vi "Add Database RTM.vi"(8 "error in":errorcluster, 11 "Node Ptr":u64 format="%.0x") -> (0 "error out":errorcluster)   [LabVIEW 2020, in "Communication Bus Template System Explorer.lvlib"]
doc: "This VI runs when the Add Database run-time menu is chosen. It allows the user to choose a database file and rename the database if they want a name other than the file name."
uses:
  Communication Bus Template System Explorer.lvlib
  Types/Path Control.ctl
  Types/Browse Button.ctl
  Shared/Constants.vi
  <vilib>/NI VeriStand/Custom Device API/Set Item Property (Path).vi
  Shared/Communication Bus Template Shared.lvlib
  <vilib>/NI VeriStand/Custom Device Tools/Custom Device Utility Library/Custom Device Utility Library.lvlib
  <vilib>/NI VeriStand/Custom Device API/Custom Device API.lvlib
panel:
  in  "Path":T1
  in  "Database Name":string
  in  "Help":bool
  in  "Cancel":bool
  in  "OK":bool
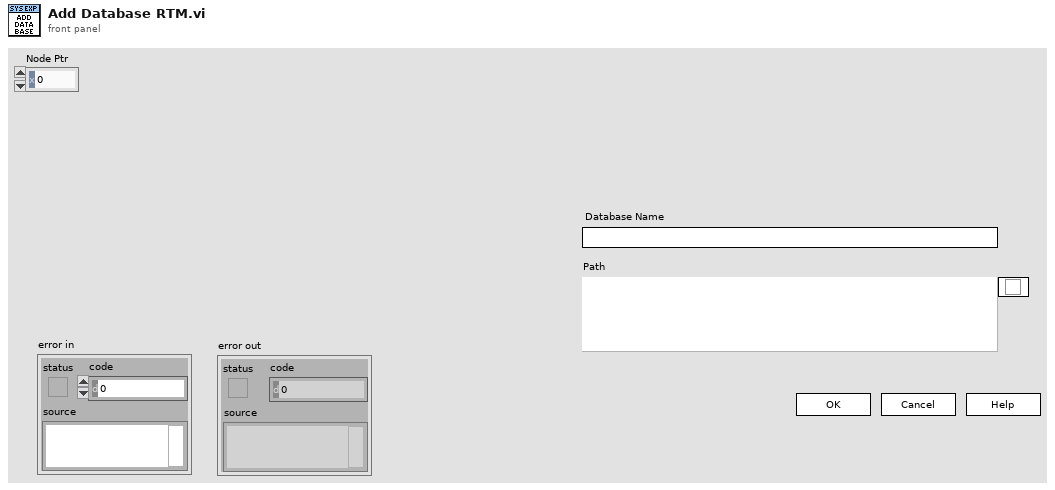
[diagram p1: front panel]
types:
  T1 = typedef "Communication Bus Template System Explorer.lvlib/Path Control.ctl" = cluster{"Path":path, "Browse":T2}
  T2 = typedef "Communication Bus Template System Explorer.lvlib/Browse Button.ctl" = bool
  T3 = cluster{"Database Name":string, "Database Path":path, "Node Ptr":u64}
  T4 = typedef "Custom Device API.lvlib/Custom Device Item Ref.ctl" = u64
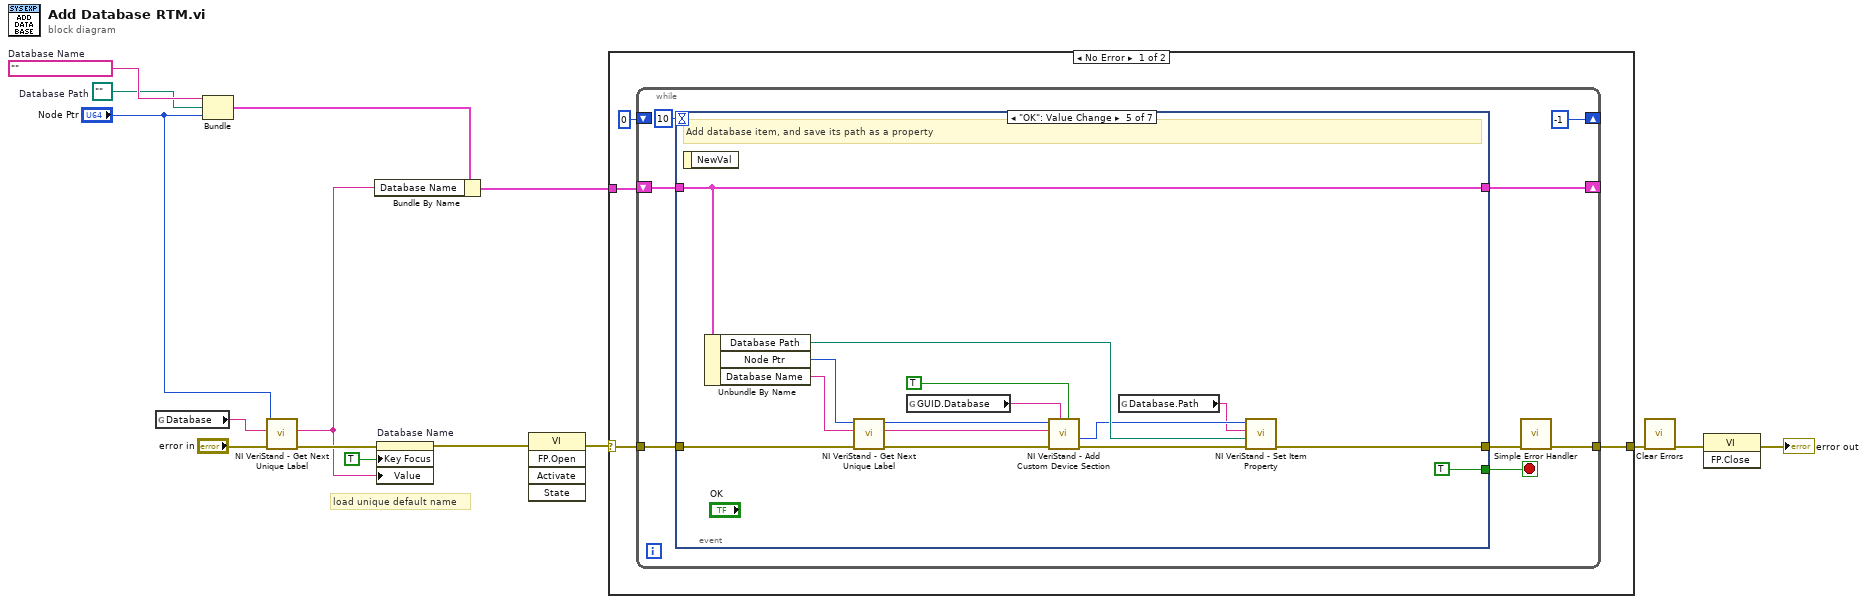
[diagram p0: block diagram]
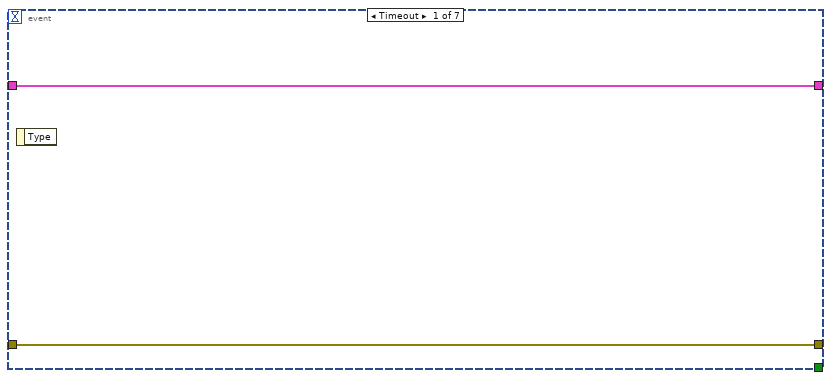
[diagram p2: hidden frame]
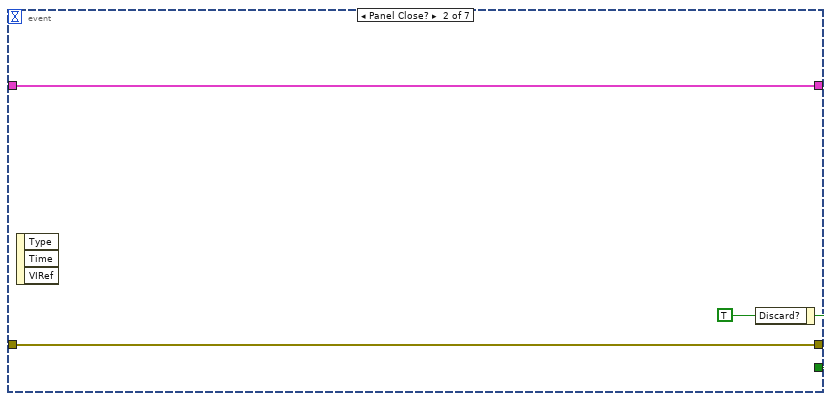
[diagram p3: hidden frame]
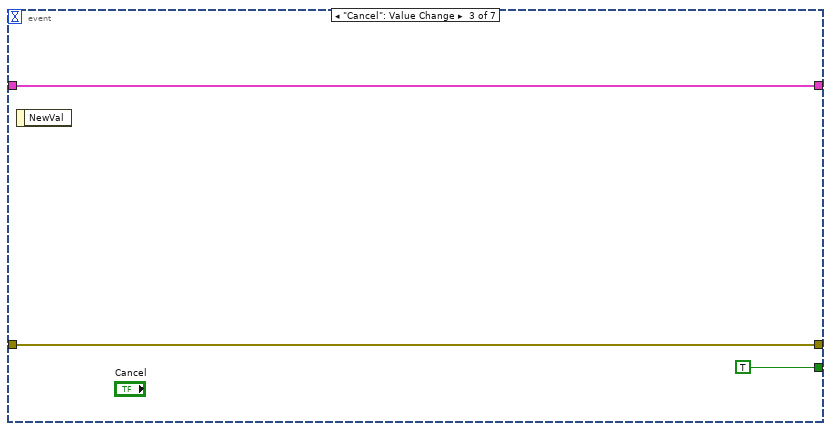
[diagram p4: hidden frame]
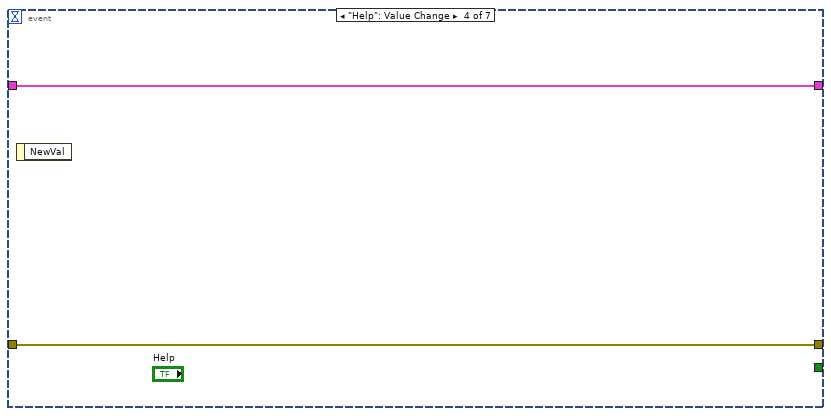
[diagram p5: hidden frame]
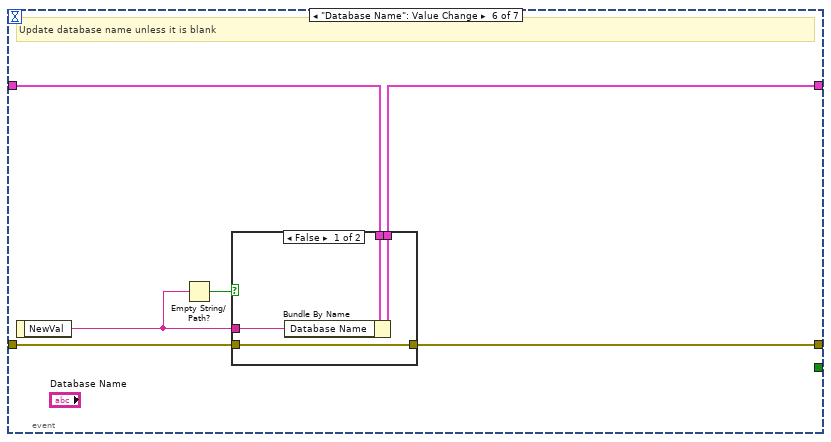
[diagram p6: hidden frame]
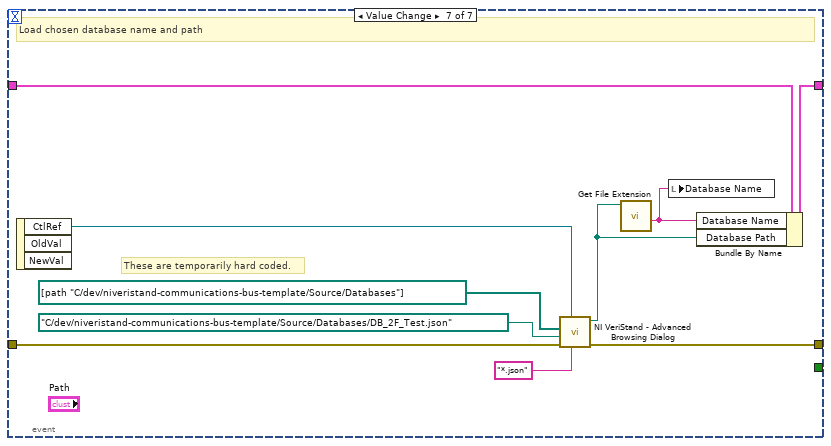
[diagram p8: hidden frame]
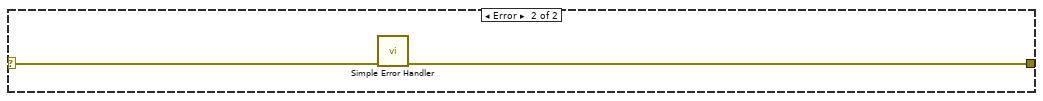
[diagram p9: hidden frame]
diagram:
  w1 = path ""  # Database Path
  w2 = ""  # Database Name
  # "load unique default name"
  n1 = global read "Constants.vi" "Database"() -> (w5:string)
  n2 = Bundle("Database Name"=w2, "Database Path"=w1, "Node Ptr"="Node Ptr") -> (w4:T3)  [unwired: 1 in]
  n3 = call <vilib>:"NI VeriStand - Get Next Unique Label.vi"("error in (no error)"="error in", "Label"=w5, "Parent Ref in"="Node Ptr") -> ("error out"=w7:errorcluster, "Label out"=w6:string)  [unwired: 5 in, 2 out]
  n4 = Bundle By Name(cluster=w4, "Database Name"=w6) -> (w13:T3)
  n5 = property on="Database Name" class="Str"(error in=w7, "Key Focus"=TRUE, "Value"=w6) -> (error out=w12:errorcluster)  [unwired: 1 in, 1 out]
  n6 = invoke class="VI" method="FP.Open"(error in=w12) -> (error out=w11:errorcluster)  [unwired: 4 in, 4 out]
  n7 = case shown="No Error" w11 {
    selector: w11 -> [w19 w76]
    tunnel: [w18 w75] -> w14
    tunnel: w13 -> [w16 _]
    frame No Error {
      n8 = while {
        tunnel: w19 -> [w27]
        tunnel: [w25] -> w18
        shift-right: [-1] -> _
        shift-left: 0 -> [_]
        shift-right: [w21] -> _
        shift-left: w16 -> [w22]
        stop <- w24 stop-if-true
        n9 = event shown="[4] \"OK\": Value Change" {
          selector: _ -> [_ _ _ _ _ _ _]
          dyn-events: _ -> [_ _ _ _ _ _ _]
          timeout: 10 -> [_ _ _ _ _ _ _]
          tunnel: [w29 w32 w34 w37 w39 w57 w69] -> w26
          tunnel: w27 -> [w29 w32 w34 w37 w48 w58 w73]
          tunnel: [_ w31 TRUE ("Discard?") _ TRUE ("Discard?") _ _] -> w24
          tunnel: w22 -> [w28 w30 w33 w36 w45 w54 w67]
          tunnel: [w28 w30 w33 w36 w45 w53 w68] -> w21
          event Timeout {
            n10 = event-data() -> ()  [unwired: 1 in, 1 out]
          }
          event Panel Close? {
            w31 = TRUE ("Discard?")
            n11 = event-data() -> ()  [unwired: 1 in, 3 out]
            n12 = event-data("Discard?"=w31) -> ()  [unwired: 1 in, 1 out]
          }
          event "Cancel": Value Change {
            n13 = event-data() -> ()  [unwired: 1 in, 1 out]
          }
          event "Help": Value Change {
            n14 = event-data() -> ()  [unwired: 1 in, 1 out]
          }
          event "OK": Value Change {
            # "Add database item, and save its path as a property"
            n15 = event-data() -> ()  [unwired: 1 in, 1 out]
            n16 = Unbundle By Name(w45) -> ("Database Path"=w41:path, "Node Ptr"=w44:u64, "Database Name"=w43:string)
            n17 = call <vilib>:"NI VeriStand - Get Next Unique Label.vi"("error in (no error)"=w48, "Label"=w43, "Parent Ref in"=w44) -> ("error out"=w49:errorcluster, "Label out"=w46:string, "Parent Ref dup"=w47:T4)  [unwired: 5 in, 1 out]
            n18 = global read "Constants.vi" "GUID.Database"() -> (w50:string)
            n19 = call <vilib>:"NI VeriStand - Add Custom Device Section.vi"("Highlight? (F)"=TRUE, "GUID (Default Section)"=w50, "error in (no error)"=w49, "Section Name"=w46, "Parent Ref in"=w47) -> ("error out"=w42:errorcluster, "Section Ptr"=w40:T4)  [unwired: 3 in, 2 out]
            n20 = global read "Constants.vi" "Database.Path"() -> (w38:string)
            n21 = call-poly <vilib>:"NI VeriStand - Set Item Property.vi"("error in (no error)"=w42, "Value"=w41, "Property Name"=w38, "Item Ref in"=w40) -> ("error out"=w39:errorcluster)  [unwired: 5 in, 2 out]
          }
          event "Database Name": Value Change {
            # "Update database name unless it is blank"
            n22 = event-data() -> ("NewVal"=w55:string)  [unwired: 1 in]
            n23 = Empty String/Path?(string/path=w55) -> (empty?=w56:bool)
            n24 = case shown="False" w56 {
              tunnel: w58 -> [w62 w64]
              tunnel: w55 -> [w60 _]
              tunnel: [w62 w64] -> w57
              tunnel: w54 -> [w61 w63]
              tunnel: [w59 w63] -> w53
              frame False {
                n25 = Bundle By Name(cluster=w61, "Database Name"=w60) -> (w59:T3)
              }
              frame True {
              }
            }
          }
          event Value Change {
            # "These are temporarily hard coded."
            # "Load chosen database name and path"
            n26 = event-data() -> ("CtlRef"=w74:refnum<vi>)  [unwired: 1 in, 2 out]
            n27 = call <vilib>:"NI VeriStand - Advanced Browsing Dialog.vi"("File Pattern"="*.json", "CtlRef"=w74, "error in (no error)"=w73, "Most recent path"=path "C:/dev/niveristand-communications-bus-template/Source/Databases/DB_2F_Test.json", "Paths"=path[] [path "C:/dev/niveristand-communications-bus-template/Source/Databases"]) -> ("error out"=w69:errorcluster, "Selected file"=w65:path)  [unwired: 3 in, 2 out]
            n28 = call <vilib>:"Get File Extension.vi"("file"=w65) -> ("filename without extension"=w66:string)  [unwired: 6 in, 4 out]
            n29 = local write "Database Name"(w66) -> ()
            n30 = Bundle By Name(cluster=w67, "Database Name"=w66, "Database Path"=w65) -> (w68:T3)
          }
        }
        n31 = call <vilib>:"Simple Error Handler.vi"("error in (no error)"=w26) -> ("error out"=w25:errorcluster)  [unwired: 4 in, 4 out]
      }
    }
    frame Error {
      n32 = call <vilib>:"Simple Error Handler.vi"("error in (no error)"=w76) -> ("error out"=w75:errorcluster)  [unwired: 4 in, 4 out]
    }
  }
  n33 = call <vilib>:"Clear Errors.vi"("error in (no error)"=w14) -> ("error out"=w10:errorcluster)  [unwired: 5 in, 1 out]
  n34 = invoke class="VI" method="FP.Close"(error in=w10) -> (error out=→"error out":errorcluster)  [unwired: 2 in, 2 out]
